vi "Setpoints.vi"() -> (13 "Arm Hic up":dbl, 14 "Arm Base Offset":dbl, 15 "Climb position":dbl, 16 "Sally Door":dbl, 17 "Portcullis up position":dbl, 18 "Drawbridge position":dbl, 19 "Drive position":dbl)   [LabVIEW 2015]
uses:
  <vilib>/Utility/file.llb/Read Delimited Spreadsheet (DBL).vi
panel:
  out "Setpoints File Selected":string
  in  "File Number\nto Select":i32
  out "Number of Setpoint Files":i64
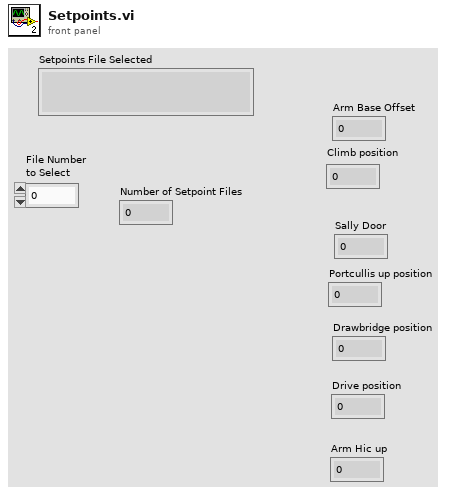
[diagram p1: front panel]
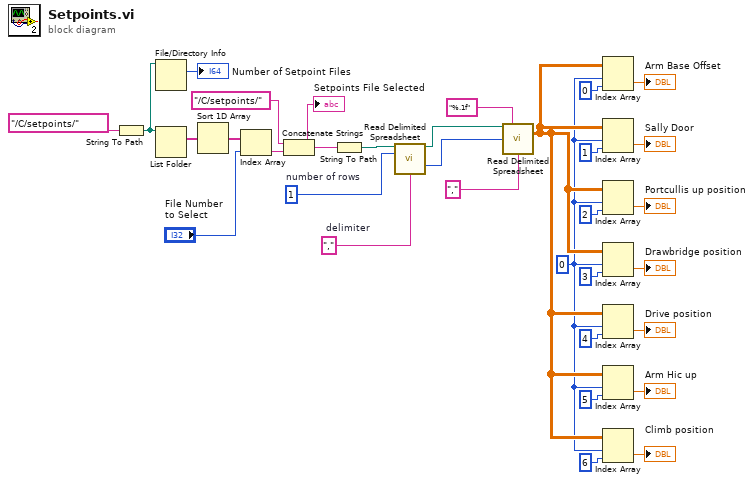
[diagram p0: block diagram]
diagram:
  w16 = 1  # number of rows
  w17 = ","  # delimiter
  w1 = 0 ("index (col)")
  n1 = String To Path(string="/C/setpoints/") -> (path=w25:path)
  n2 = File/Directory Info(path=w25) -> (size=→"Number of Setpoint Files":i64)  [unwired: 1 in, 6 out]
  n3 = List Folder(path=w25) -> (filenames=w26:string[])  [unwired: 1 in, 5 out]
  n4 = Sort 1D Array(array=w26) -> (sorted array=w28:string[])
  n5 = Index Array(array=w28, index="File Number\nto Select") -> (element=w23:string)
  n6 = Concatenate Strings("/C/setpoints/" ("string"), w23) -> (w30:string)
  "Setpoints File Selected" <- w30
  n7 = String To Path(string=w30) -> (path=w15:path)
  n8 = call-poly <vilib>:"Read Delimited Spreadsheet.vi"("file path (dialog if empty)"=w15, "number of rows (all:-1)"=w16, "delimiter (\\t)"=w17) -> ("new file path (Not A Path if cancelled)"=w14:path, "mark after read (chars.)"=w13:i32)  [unwired: 7 in, 4 out]
  n9 = call-poly <vilib>:"Read Delimited Spreadsheet.vi"("file path (dialog if empty)"=w14, "format (%.3f)"="%.1f", "start of read offset (chars.:0)"=w13, "delimiter (\\t)"="," ("delimiter (\\t)")) -> ("all rows"=w2:dbl[][])  [unwired: 6 in, 5 out]
  n10 = Index Array(array=w2, index (row)=w1, index (col)=0 ("disabled index (col)")) -> (element=→"Arm Base Offset":dbl)
  n11 = Index Array(array=w2, index (row)=w1, index (col)=1 ("disabled index (col)")) -> (element=→"Sally Door":dbl)
  n12 = Index Array(array=w2, index (row)=w1, index (col)=2 ("disabled index (col)")) -> (element=→"Portcullis up position":dbl)
  n13 = Index Array(array=w2, index (row)=w1, index (col)=3 ("disabled index (col)")) -> (element=→"Drawbridge position":dbl)
  n14 = Index Array(array=w2, index (row)=w1, index (col)=4 ("disabled index (col)")) -> (element=→"Drive position":dbl)
  n15 = Index Array(array=w2, index (row)=w1, index (col)=5 ("disabled index (col)")) -> (element=→"Arm Hic up":dbl)
  n16 = Index Array(array=w2, index (row)=w1, index (col)=6 ("disabled index (col)")) -> (element=→"Climb position":dbl)
